vi "DayNEW.vi"(8 "error in (no error)":errorcluster, 11 "Archive in":refnum<class "Archive.lvclass">) -> (0 "error out":errorcluster, 2 "NewDay":bool, 3 "Archive out":refnum<class "Archive.lvclass">)   [LabVIEW 2010, in "Archive.lvclass"]
uses:
  Archive.lvclass
  Archive.lvclass/Archive.ctl
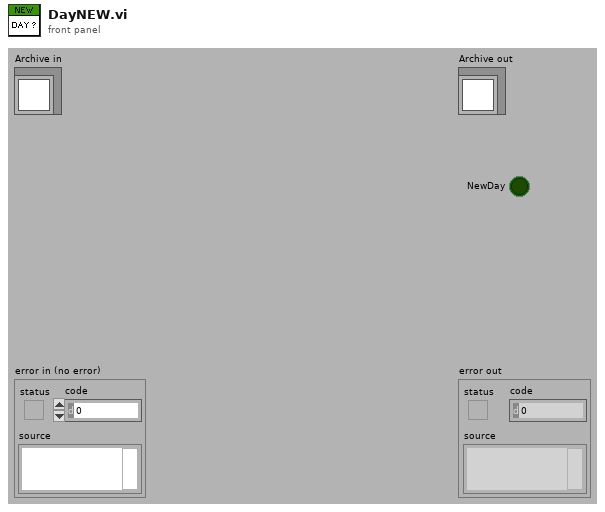
[diagram p1: front panel]
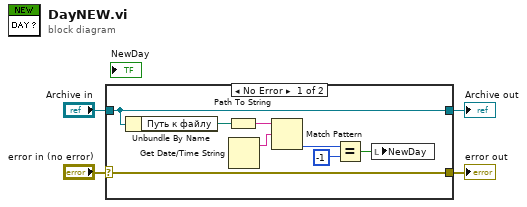
[diagram p0: block diagram]
diagram:
  n1 = case shown="No Error" "error in (no error)" {
    selector: "error in (no error)" -> [w12 w14]
    tunnel: [w12 w14] -> w3
    tunnel: [w7 w13] -> w1
    tunnel: "Archive in" -> [w7 w13]
    frame No Error {
      n2 = Unbundle By Name(w7) -> ("Путь к файлу"=w6:path)
      n3 = Path To String(path=w6) -> (string=w10:string)
      n4 = Get Date/Time String() -> (date string=w11:string)  [unwired: 3 in, 1 out]
      n5 = Match Pattern(string=w10, regular expression=w11) -> (offset past match=w9:i32)  [unwired: 1 in, 3 out]
      n6 = Equal?(x=w9, y=-1) -> (x = y?=w5:bool)
      n7 = local write "NewDay"(w5) -> ()
    }
    frame Error {
    }
  }
  "error out" <- w3
  "Archive out" <- w1
